vi "GetBaseFileName.vi"(8 "error in":errorcluster, 11 "Datawarehouse in":refnum<class "Datawarehouse.lvclass">) -> (0 "error out":errorcluster, 2 "BaseFileName":string, 3 "Datawarehouse out":refnum<class "Datawarehouse.lvclass">)   [LabVIEW 2021, in "ProligentXMLGenerator.lvlib" / "Datawarehouse.lvclass"]
doc: "Base file name used to create the full file name.\n\nThe full file name is composed of a \"Proligent_\" prefix and the \".xml\" extension."
uses:
  Datawarehouse.lvclass
  Datawarehouse.lvclass/Datawarehouse.ctl
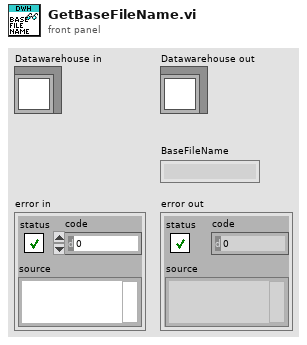
[diagram p1: front panel]
types:
  T1 = typedef "ProligentXMLGenerator.lvlib/Datawarehouse.lvclass/Data.ctl" = cluster{"DestinationFolder":path, "BaseFileName":string, "Document":refnum<k20>, "Defects":refnum<class "Defect.lvclass">[], "TopProcessRuns":refnum<class "ProcessRun.lvclass">[], "ProductUnits":refnum<class "ProductUnit.lvclass">[], "GenerationTime":refnum<class "DateTime.lvclass">, "DataSourceFingerprint":refnum<class "NonEmptyString_448.lvclass">, "IntegrationMetaData":refnum<class "NonEmptyString_2000.lvclass">, "TimeZoneInfoId":string}
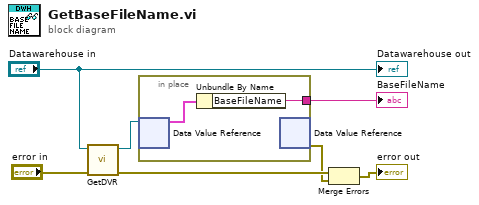
[diagram p0: block diagram]
diagram:
  n1 = call "GetDVR.vi"("error in"="error in", "Datawarehouse"="Datawarehouse in") -> ("error out"=w7:errorcluster, "DVRReference"=w5:refnum<data-value>)  [unwired: 8 in]
  n2 = in-place "In Place Element Structure" {
    in-place-border: [w8] -> w4
    n3 = in-place-dvr #1(w5) -> (w9:T1)  [unwired: 1 out]
    n4 = Unbundle By Name(w9) -> ("BaseFileName"=w8:string)
    n5 = in-place-dvr #1() -> (w6:errorcluster)  [unwired: 1 in, 1 out]
  }
  "BaseFileName" <- w4
  n6 = Merge Errors(w7, w6) -> (→"error out":errorcluster)
  "Datawarehouse out" <- "Datawarehouse in"
